vi "Servo Motors Control.vi"   [LabVIEW 2014]
uses:
  QwaveSys_Interface/QwaveSys_Interface.lvlib
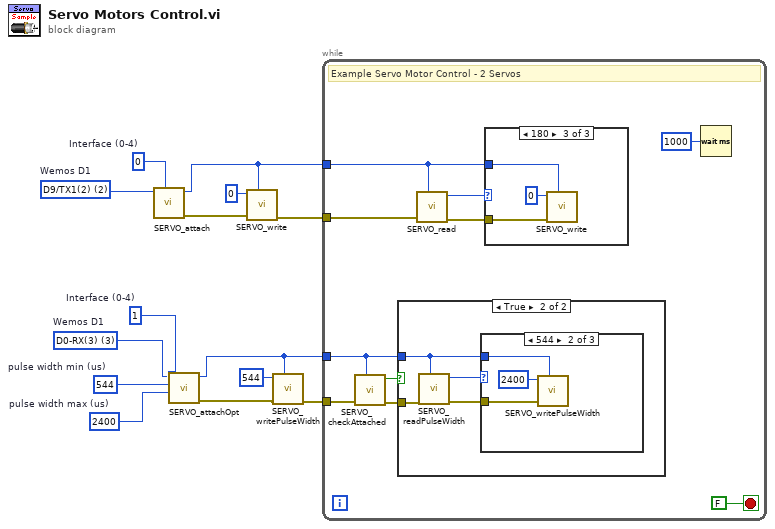
[diagram p0: block diagram]
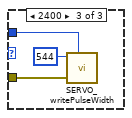
[diagram p4: hidden frame]
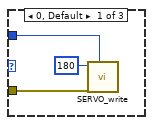
[diagram p5: hidden frame]
diagram:
  w3 = u8 3 items=["D0-RX(3)"=3, "D1-TX(1)"=1, "D2(16)"=16, "D3/D15/SCL(5)"=5, "D4/D14/SDA(4)"=4, "D5/D13/SCK(14)-(LED)"=14, "D6/D12/MISO(12)"=12, "D7/D11/MOSI(13)"=13, "D8(0)"=0, "D9/TX1(2)"=2, "D10/SS (15)"=15, "ADC0,(17)"=17]  # Wemos D1
  w4 = u8 2 items=["D0-RX(3)"=3, "D1-TX(1)"=1, "D2(16)"=16, "D3/D15/SCL(5)"=5, "D4/D14/SDA(4)"=4, "D5/D13/SCK(14)-(LED)"=14, "D6/D12/MISO(12)"=12, "D7/D11/MOSI(13)"=13, "D8(0)"=0, "D9/TX1(2)"=2, "D10/SS (15)"=15, "ADC0,(17)"=17]  # Wemos D1
  w2 = u16 2400  # pulse width max (us)
  w1 = u16 544  # pulse width min (us)
  w5 = u8 1  # Interface (0-4)
  w14 = u8 0  # Interface (0-4)
  n1 = call "SERVO_attach.vi"("Interface (0-4)"=w14, "PIN"=w4) -> ("error out"=w13:errorcluster, "Instance"=w10:u8)  [unwired: 8 in]
  n2 = call "SERVO_attachOpt.vi"("Interface (0-4)"=w5, "pulse width max (us)"=w2, "pulse width min (us)"=w1, "PIN"=w3) -> ("error out"=w8:errorcluster, "Instance"=w6:u8)  [unwired: 6 in]
  n3 = call "SERVO_write.vi"("Instance"=w10, "error in (no error)"=w13, "angle"=u8 0) -> ("error out"=w11:errorcluster)  [unwired: 8 in]
  n4 = call "SERVO_writePulseWidth.vi"("Instance"=w6, "error in (no error)"=w8, "pulse width (us)"=u16 544) -> ("error out"=w9:errorcluster)  [unwired: 8 in]
  n5 = while {
    tunnel: w11 -> [w24]
    tunnel: w10 -> [w23]
    tunnel: w9 -> [w18]
    tunnel: w6 -> [w17]
    stop <- FALSE stop-if-true
    # "Example Servo Motor Control - 2 Servos"
    n6 = call "SERVO_checkAttached.vi"("Instance"=w17, "error in (no error)"=w18) -> ("error out"=w16:errorcluster, "attached"=w15:bool)  [unwired: 8 in]
    n7 = case shown="True" w15 {
      tunnel: w17 -> [_ w26]
      tunnel: w16 -> [_ w25]
      frame False {
      }
      frame True {
        n8 = call "SERVO_readPulseWidth.vi"("Instance"=w26, "error in (no error)"=w25) -> ("error out"=w28:errorcluster, "pulse width (us)"=w27:u16)  [unwired: 8 in]
        n9 = case shown="544" w27 {
          tunnel: w28 -> [_ w31 w33]
          tunnel: w26 -> [_ w30 w32]
          frame 0, Default {
          }
          frame 544 {
            n10 = call "SERVO_writePulseWidth.vi"("Instance"=w30, "error in (no error)"=w31, "pulse width (us)"=u16 2400) -> ()  [unwired: 8 in, 1 out]
          }
          frame 2400 {
            n11 = call "SERVO_writePulseWidth.vi"("Instance"=w32, "error in (no error)"=w33, "pulse width (us)"=u16 544) -> ()  [unwired: 8 in, 1 out]
          }
        }
      }
    }
    n12 = call "SERVO_read.vi"("Instance"=w23, "error in (no error)"=w24) -> ("error out"=w20:errorcluster, "angle"=w21:u8)  [unwired: 8 in]
    n13 = case shown="180" w21 {
      tunnel: w20 -> [w37 _ w40]
      tunnel: w23 -> [w35 _ w38]
      frame 0, Default {
        n14 = call "SERVO_write.vi"("Instance"=w35, "error in (no error)"=w37, "angle"=u8 180) -> ()  [unwired: 8 in, 1 out]
      }
      frame 1..179 {
      }
      frame 180 {
        n15 = call "SERVO_write.vi"("Instance"=w38, "error in (no error)"=w40, "angle"=u8 0) -> ()  [unwired: 8 in, 1 out]
      }
    }
    n16 = Wait (ms)(milliseconds to wait=u32 1000) -> ()  [unwired: 1 out]
  }
